vi "FinishMessage.vi"(6 "error in":errorcluster, 9 "RasPi Compiler in":refnum<class "RasPi Compiler.lvclass">) -> (0 "error out":errorcluster, 3 "RasPi Compiler out":refnum<class "RasPi Compiler.lvclass">)   [LabVIEW 2014, in "RasPi Compiler.lvclass"]
uses:
  RasPi Compiler.lvclass
  RasPi Compiler.lvclass/RasPi Compiler.ctl
  RasPi_Services/MessageBox/MessageBox.lvclass
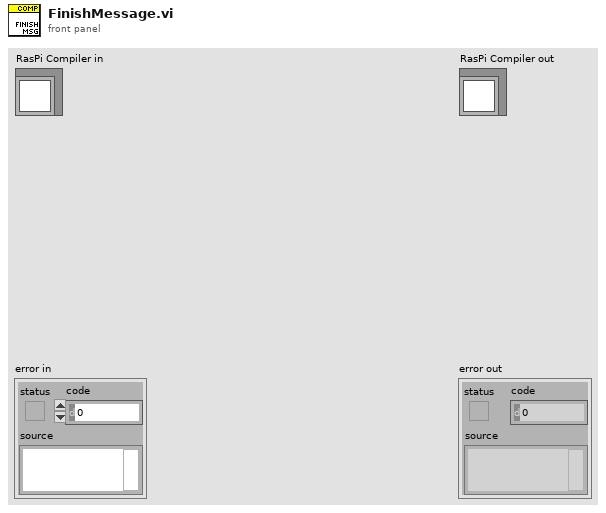
[diagram p1: front panel]
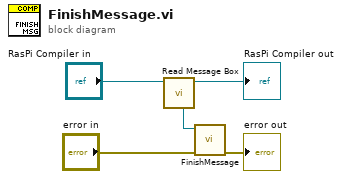
[diagram p0: block diagram]
diagram:
  n1 = call "Read Message Box.vi"("RasPi Compiler in"="RasPi Compiler in") -> ("RasPi Compiler out"=→"RasPi Compiler out":refnum<class "RasPi Compiler.lvclass">, "Message Box"=w3:refnum<class "MessageBox.lvclass">)  [unwired: 7 in]
  n2 = call "FinishMessage.vi"("error in"="error in", "MessageBox in"=w3) -> ("error out"=→"error out":errorcluster)  [unwired: 6 in, 1 out]
